vi "ErrorHandler.vi"(8 "error in (no error)":errorcluster, 11 "Queue in":refnum<queue>) -> (0 "error out":errorcluster)   [LabVIEW 2019, in "Prueba09.lvclass"]
uses:
  Prueba09.lvclass
  Controles/MessageP09.ctl
  Controles/Estados_P09.ctl
  <vilib>/ErrorRing/Error Ring.xnode
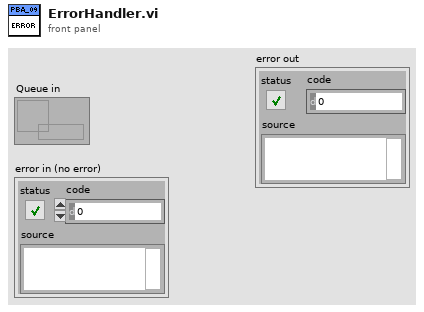
[diagram p1: front panel]
types:
  T1 = typedef "Prueba09.lvclass/Estados_P09.ctl" = enum16{"Error", "DetieneInstrumentos", "InicializarInstrumentos", "LeerArchivoConfiguracion", "inicio", "configurarTabla", "FrecAmp1", "FrecAmp2", "FrecAmp3", "iniciarGEN", "iniciaGEN_Peak", "detenerGEN", "guardaVref", "guardaVref2", "monitoreo", "peakRefer", "ingresaMediciones", "guardaMediciones", "cumplimiento", "listo_evaluar", "evaluar", "final", "salir"}
  T2 = typedef "Prueba09.lvclass/MessageP09.ctl" = cluster{"Estados":T1, "Data":variant}
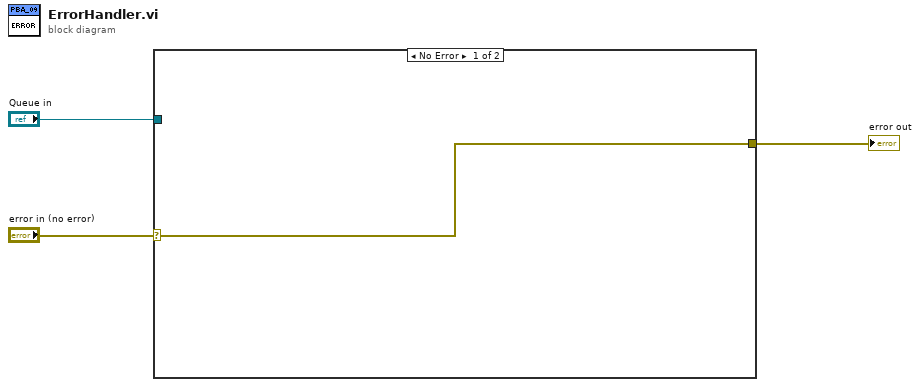
[diagram p0: block diagram]
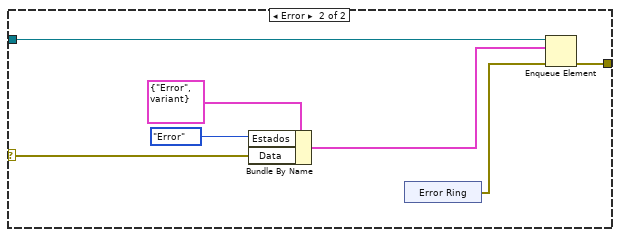
[diagram p2: hidden frame]
diagram:
  n1 = case shown="No Error" "error in (no error)" {
    selector: "error in (no error)" -> [w4 w8]
    tunnel: "Queue in" -> [_ w10]
    tunnel: [w4 w11] -> w1
    frame No Error {
    }
    frame Error {
      n2 = Bundle By Name(cluster=T2 {"Estados"=enum."Error", "Data"=variant} ("MessageP08"), "Estados"=Estados_P09."Error", "Data"=w8) -> (w6:T2)
      n3 = xnode "Error Ring"() -> ("error out"=w5:errorcluster)
      n4 = Enqueue Element(queue=w10, element=w6, error in (no error)=w5) -> (error out=w11:errorcluster)  [unwired: 1 in, 2 out]
    }
  }
  "error out" <- w1
